vi "GetTimeStamp.vi"(0 "Image":T1, 1 "error in (no error)":errorcluster) -> (2 "Image (duplicate)":T1, 3 "Timestamp":timestamp, 4 "Time(ms)":dbl, 5 "error out":errorcluster)   [LabVIEW 2021]
uses:
  <vilib>/vision/Image Controls.llb/IMAQ Image.ctl
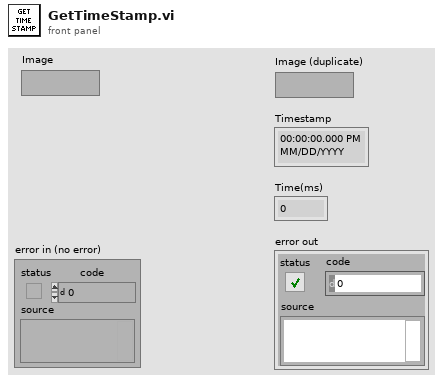
[diagram p1: front panel]
types:
  T1 = typedef "IMAQ Image.ctl" = refnum<image>
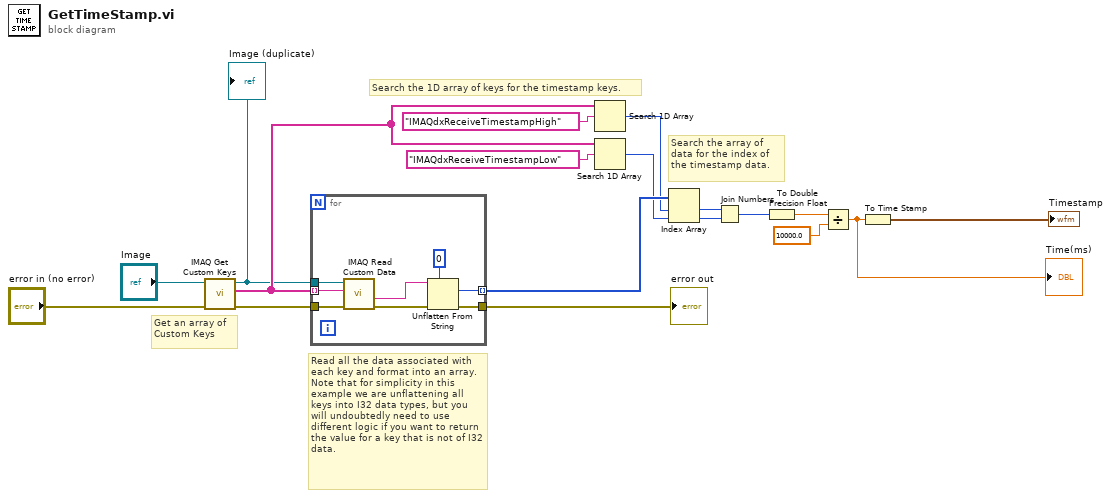
[diagram p0: block diagram]
diagram:
  # "Search the array of data for the index of the timestamp data."
  # "Search the 1D array of keys for the timestamp keys."
  # "Read all the data associated with each key and format into an array. Note that for simplicity in this example we are unflattening all keys into I32 data types, but you will undoubtedly need to use different logic if you want to return the value for a key that is not of I32 data."
  # "Get an array of Custom Keys"
  n1 = call "IMAQ Get Custom Keys"("error in (no error)"="error in (no error)", "Image"="Image") -> ("error out"=w18:errorcluster, "Keys"=w12:string[], "Image (duplicate)"=w6:T1)  [unwired: 6 in, 1 out]
  "Image (duplicate)" <- w6
  n2 = for {
    tunnel: w6 -> [w26]
    tunnel: w18 -> [w25]
    tunnel: [w24] -> w1
    tunnel: w12 -> [w23] mode=indexing
    tunnel: [w22] -> w17 mode=indexing
    n3 = call "IMAQ Read Custom Data"("error in (no error)"=w25, "Key"=w23, "Image"=w26) -> ("error out"=w21:errorcluster, "Custom Data Out"=w20:string)  [unwired: 6 in, 1 out]
    n4 = Unflatten From String(type=0, binary string=w20, error in (no error)=w21) -> (value=w22:i32, error out=w24:errorcluster)  [unwired: 2 in, 1 out]
  }
  "error out" <- w1
  n5 = Search 1D Array(1D array=w12, element="IMAQdxReceiveTimestampHigh") -> (index of element=w13:i32)  [unwired: 1 in]
  n6 = Search 1D Array(1D array=w12, element="IMAQdxReceiveTimestampLow") -> (index of element=w14:i32)  [unwired: 1 in]
  n7 = Index Array(array=w17, index #1=w13, index #2=w14) -> (element #1=w10:i32, element #2=w11:i32)
  n8 = Join Numbers(hi=w10, lo=w11) -> ((hi.lo)=w9:u64)
  n9 = To Double Precision Float(number=w9) -> (double precision float=w8:dbl)
  n10 = Divide(x=w8, y=10000.0) -> (x/y=w5:dbl)
  "Time(ms)" <- w5
  n11 = To Time Stamp(1:w5) -> (0:→"Timestamp":timestamp)
